vi "Close.vi"(8 "error in (no error)":errorcluster, 11 "Data in":refnum<class "Fault-Injection_I64.lvclass">) -> (0 "error out":errorcluster, 3 "Data out":refnum<class "Fault-Injection_I64.lvclass">)   [LabVIEW 2021, in "Fault-Injection_I64.lvclass"]
doc: "Abstract Data Classes 2.1.1.12\nTim Streeter - TSA\nCopyright (c) 2024, TSA"
uses:
  Fault-Injection_I64.lvclass
  Fault-Injection_I64.lvclass/Fault-Injection_I64.ctl
  <vilib>/TSA/Abstract Data Classes/Abs_Types/I64 Integer/Abs_I64 Integer.lvclass
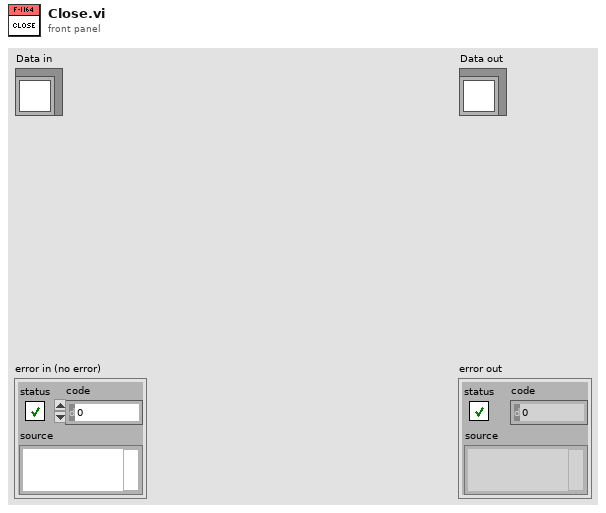
[diagram p1: front panel]
types:
  T1 = typedef "Fault-Injection_I64.lvclass/DVR Type.ctl" = cluster{"Enable":bool, "Injected Value":T2, "Value":T3}
  T2 = typedef "Fault-Injection_I64.lvclass/Value Type.ctl" = i64
  T3 = typedef "Fault-Injection_I64.lvclass/Abs Class Type.ctl" = refnum<class "Abs_I64 Integer.lvclass">
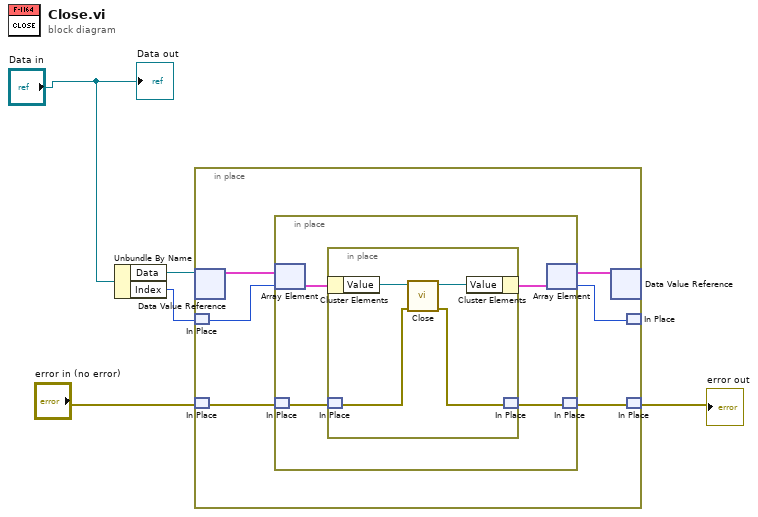
[diagram p0: block diagram]
diagram:
  n1 = Unbundle By Name("Data in") -> ("Data"=w5:refnum<data-value>, "Index"=w4:i32)
  n2 = in-place {
    n3 = in-place-dvr #1(w5) -> (w11:T1[])  [unwired: 1 out]
    n4 = in-place-match #2(w4) -> (w9:i32)
    n5 = in-place-match #3("error in (no error)") -> (w7:errorcluster)
    n6 = in-place {
      n7 = in-place-array #4(w11, w9) -> (w12:T1)
      n8 = in-place-match #5(w7) -> (w14:errorcluster)
      n9 = in-place {
        n10 = in-place-cluster #6(w12) -> ("Value"=w16:T3)
        n11 = in-place-match #7(w14) -> (w18:errorcluster)
        n12 = call-dynamic "Close.vi"("error in (no error)"=w18, "Data in"=w16) -> ("error out"=w17:errorcluster, "Data out"=w19:T3)  [unwired: 8 in]
        n13 = in-place-cluster #6("Value"=w19) -> (w15:T1)
        n14 = in-place-match #7(w17) -> (w13:errorcluster)
      }
      n15 = in-place-array #4(w15) -> (w10:T1[], w8:i32)
      n16 = in-place-match #5(w13) -> (w6:errorcluster)
    }
    n17 = in-place-dvr #1(w10) -> ()  [unwired: 2 out]
    n18 = in-place-match #2(w8) -> ()  [unwired: 1 out]
    n19 = in-place-match #3(w6) -> (→"error out":errorcluster)
  }
  "Data out" <- "Data in"
